vi "SP Calculate SYY.vi"(10 "TP Array (TXX, TXY, TYX, TYY)":cdb[](array[numeric])) -> (2 "SYY":cdb)   [LabVIEW 2011]
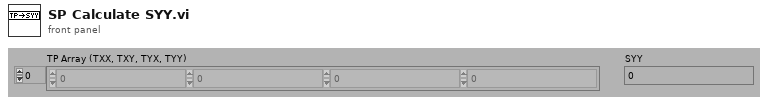
[diagram p1: front panel]
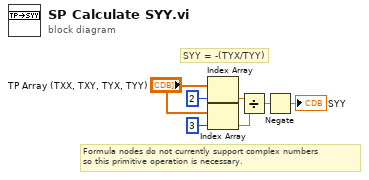
[diagram p0: block diagram]
diagram:
  # "SYY = -(TYX/TYY)"
  # "Formula nodes do not currently support complex numbers\nso this primitive operation is necessary."
  n1 = Index Array(array="TP Array (TXX, TXY, TYX, TYY)", index=2) -> (element=w2:cdb)
  n2 = Index Array(array="TP Array (TXX, TXY, TYX, TYY)", index=3) -> (element=w1:cdb)
  n3 = Divide(x=w2, y=w1) -> (x/y=w4:cdb)
  n4 = Negate(x=w4) -> (-x=→"SYY":cdb)
